vi "From JSON.vi"(8 "error in":errorcluster, 10 "File Path":path, 11 "Acquire Continuous Waveform Configuration in":refnum<class "Continuous Waveform Acq CFG.lvclass">) -> (0 "error out":errorcluster, 3 "Acquire Continuous Waveform Configuration out":refnum<class "Continuous Waveform Acq CFG.lvclass">)   [LabVIEW 2023]
uses:
  Continuous Waveform Acq CFG.lvclass
  Configuration Base/Configuration Base.lvclass/Configuration Base.ctl
  Continuous Waveform Acq CFG.lvclass/Continuous Waveform Acq CFG.ctl
  4f3f503e-35f1-485b-b93d-ab42f3a5784a.vi
  <vilib>/JDP Science/JSONtext/Next JSON Value.vi
  <vilib>/JDP Science/JSONtext/String Subset.vi
  <vilib>/JDP Science/JSONtext/Parsing/Advance past next JSON Value (inlined COPY).vi
  <vilib>/JDP Science/JSONtext/Parsing/Advance past whitespace.vi
  <vilib>/JDP Science/JSONtext/Parsing/Advance past String.vi
  <vilib>/JDP Science/JSONtext/Parsing/Advance past Number.vi
  <vilib>/JDP Science/JSONtext/Parsing/Advance past Line Ending.vi
  <vilib>/JDP Science/JSONtext/Parsing/Parse Full Path or Item Name.vi
  <vilib>/JDP Science/JSONtext/Parsing/Advance past Array.vi
  <vilib>/JDP Science/JSONtext/Parsing/Advance past Object.vi
  <vilib>/JDP Science/JSONtext/support/Error Cluster From Code.vi
  <vilib>/JDP Science/JSONtext/Offset/Find Item Locations by Path.vi
  <vilib>/JDP Science/JSONtext/JSON text to Variant.vi
  <vilib>/Utility/error.llb/Error Cluster From Error Code.vi
  Scope VISA/Configuration/Scope VISA CFG.lvclass
  <vilib>/JDP Science/JSONtext/LVClass Serializer/JSONtext LVClass Serializer.lvclass
  <vilib>/ErrorRing/Error Ring.xnode
  Configuration Base/Configuration Base.lvclass
  <vilib>/JDP Science/JSONtext/JSONtext.lvlib
  D:/git/HAL/Scope VISA/Configuration/Scope VISA CFG.lvclass
  D:/git/HAL/Configuration Base/Configuration Base.lvclass
  D:/git/HAL/Interfaces/IConfigure/IConfigure.lvclass
  D:/git/HAL/Devices/Rigol DS1054/Configurations/Acquire Conintuous Waveform/Continuous Waveform Acq CFG.lvclass
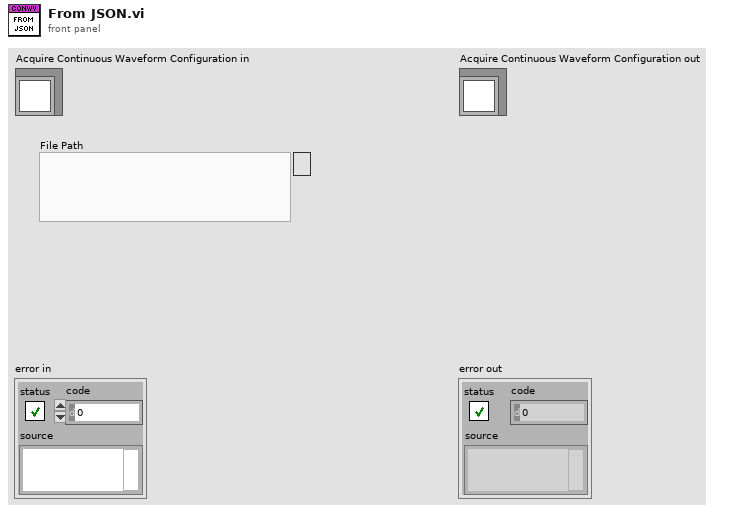
[diagram p1: front panel]
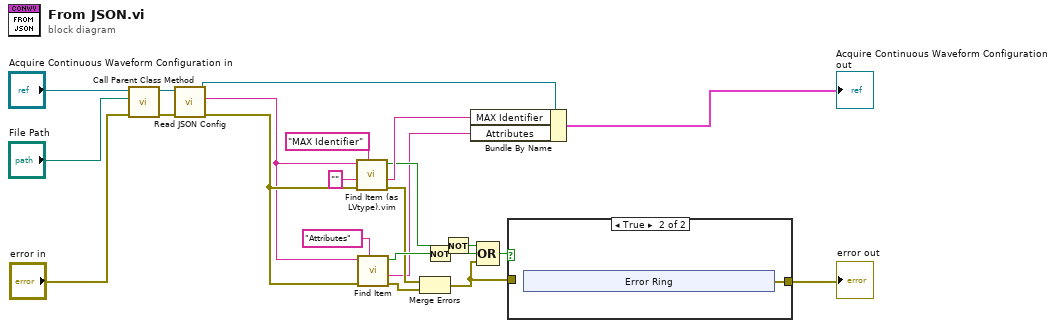
[diagram p0: block diagram]
diagram:
  n1 = call-parent "Call Parent Class Method"("error in (no error)"="error in", "JSON Config"="File Path", "Camera Config in"="Acquire Continuous Waveform Configuration in") -> ("error out"=w19:errorcluster, "Camera Config out"=w20:refnum<class "Continuous Waveform Acq CFG.lvclass">)  [unwired: 7 in]
  n2 = call "Read JSON Config.vi"("error in (no error)"=w19, "Camera Config in"=w20) -> ("error out"=w15:errorcluster, "<JSON>Config"=w14:string, "Camera Config out"=w2:refnum<class "Continuous Waveform Acq CFG.lvclass">)  [unwired: 7 in]
  n3 = call "Find Item (as LVtype).vim"("$Path or Item Name"="MAX Identifier", "error in (no error)"=w15, "Data Type and Default Value"="", "JSON"=w14) -> ("error out"=w8:errorcluster, "Data"=w16:string, "Found"=w12:bool)  [unwired: 4 in, 1 out]
  n4 = call <vilib>:"Find Item.vi"("$Path or Item Name"="Attributes", "error in (no error)"=w15, "JSON"=w14) -> ("error out"=w7:errorcluster, "<JSON>"=w3:string, "Found"=w11:bool)  [unwired: 5 in, 1 out]
  n5 = Merge Errors(w8, w7) -> (w5:errorcluster)
  n6 = Not(x=w11) -> (.not. x?=w9:bool)
  n7 = Not(x=w12) -> (.not. x?=w10:bool)
  n8 = Bundle By Name(cluster=w2, "MAX Identifier"=w16, "Attributes"=w3) -> (→"Acquire Continuous Waveform Configuration out":cluster{})
  n9 = Compound Arithmetic op=OR(w10, w9, w5) -> (w6:bool)
  n10 = case shown="True" w6 {
    tunnel: w5 -> [w24 _]
    tunnel: [w24 w25] -> w4
    frame False {
    }
    frame True {
      n11 = xnode "Error Ring"() -> ("error out"=w25:errorcluster)
    }
  }
  "error out" <- w4
